vi "test-1.vi"() -> ()   [LabVIEW 2022 SP3]
panel:
  in  "Boolean":bool
  out "Thermometer":dbl(slide) scale=0.0..100.0
  in  "Slide":dbl(slide) scale=0.0..50.0
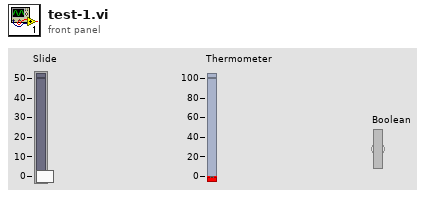
[diagram p1: front panel]
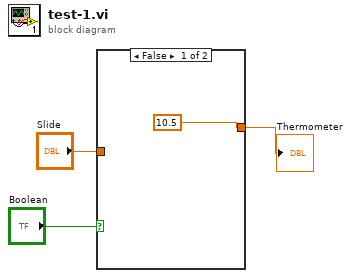
[diagram p0: block diagram]
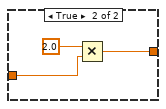
[diagram p2: hidden frame]
diagram:
  n1 = case shown="False" "Boolean" {
    tunnel: "Slide" -> [_ w7]
    tunnel: [10.5 w6] -> w2
    frame False {
    }
    frame True {
      n2 = Multiply(x=2.0, y=w7) -> (x*y=w6:dbl)
    }
  }
  "Thermometer" <- w2
